vi "Producer Loop.vi"(5 "Max delay (ms)":u32=1000, 7 "Command Array":string[](array[string])=["ABS Pos Move", "REL Pos Move", "Velocity Move"], 8 "error in (no error)":errorcluster, 9 "Motion Parameters (Min)":T1={"position"=-10000.0, "velocity"=-10000.0, "acceleration"=50000.0, "deceleration"=50000.0, "accel. jerk"=800000.0, "decel. jerk"=800000.0}, 10 "Motion Parameters (Max)":T1={"position"=10000.0, "velocity"=10000.0, "acceleration"=100000.0, "deceleration"=100000.0, "accel. jerk"=1000000.0, "decel. jerk"=1000000.0}, 11 "Axis Array":refnum<k21>[](array[refnum])=["Axis 1", "Axis 2", "Axis 3", "Axis 4", "Axis 5", "Axis 6", "Axis 7", "Axis 8"]) -> (0 "error out":errorcluster)   [LabVIEW 2013]
doc: "Generates motion commands. This is an reentrant VI."
uses:
  EMC API/EMC_Typedef_Motor_Parameters.ctl
  Functional_Global/Typedef_Message_Queue_Action.ctl
  Globals/Global Stop.vi
  support/Message Queue/Message Queue.lvlib
panel:
  out "Iterations":i32
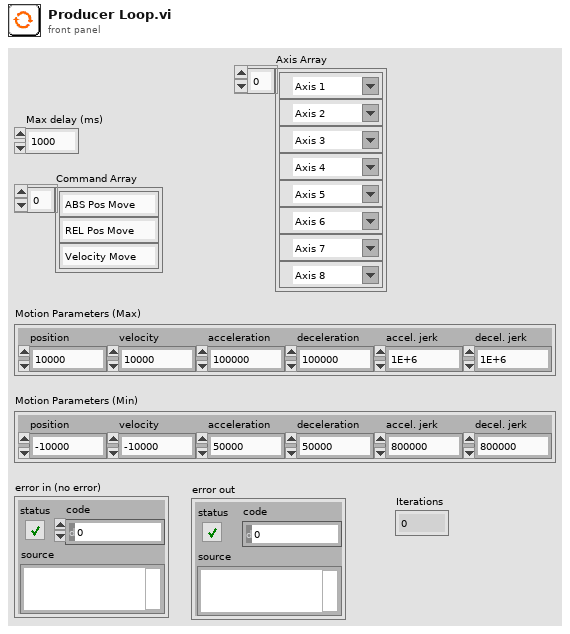
[diagram p1: front panel]
types:
  T1 = typedef "EMC_Typedef_Motor_Parameters.ctl" = cluster{"position":dbl, "velocity":dbl, "acceleration":dbl, "deceleration":dbl, "accel. jerk":dbl, "decel. jerk":dbl}
  T2 = typedef "Typedef_Message_Queue_Action.ctl" = enum16{"Init MQueue", "Get MQueue Ref", "Close MQueue"}
  T3 = typedef "Typedef_Motor_Message.ctl" = cluster{"Axis":refnum<k21>, "Motion Parameters":T1}
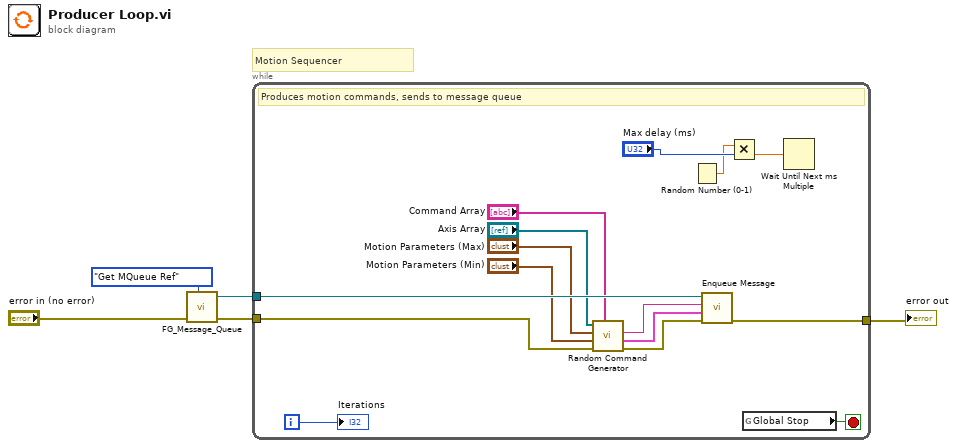
[diagram p0: block diagram]
diagram:
  # "Motion Sequencer"
  n1 = call "FG_Message_Queue.vi"("Action"=Typedef_Message_Queue_Action."Get MQueue Ref", "error in"="error in (no error)") -> ("error out"=w4:errorcluster, "Message Queue"=w3:refnum<queue>)  [unwired: 8 in]
  n2 = while {
    tunnel: w3 -> [w18]
    tunnel: [w20] -> w1
    tunnel: w4 -> [w19]
    i -> [w17]
    stop <- w11 stop-if-true
    # "Produces motion commands, sends to message queue"
    n3 = call "Random Command Generator.vi"("Command Array"="Command Array", "error in (no error)"=w19, "Motion Parameters (Min)"="Motion Parameters (Min)", "Motion Parameters (Max)"="Motion Parameters (Max)", "Axis Resources"="Axis Array") -> ("error out"=w16:errorcluster, "Motor_Message"=w14:T3, "Command Out"=w15:string)  [unwired: 4 in]
    n4 = Random Number (0-1)() -> (number: 0 to 1=w6:dbl)
    n5 = call "Enqueue Message.vi"("error in (no error)"=w16, "Message Data"=w14, "Message"=w15, "Message Queue"=w18) -> ("error out"=w20:errorcluster)  [unwired: 6 in, 1 out]
    n6 = Multiply(x=w6, y="Max delay (ms)") -> (x*y=w7:dbl)
    n7 = global read "Global Stop.vi" "Global Stop"() -> (w11:bool)
    n8 = Wait Until Next ms Multiple(millisecond multiple=w7) -> ()  [unwired: 1 out]
    "Iterations" <- w17
  }
  "error out" <- w1
